vi "Review Results.vi"(0 "Cal Results":string, 5 "Request Message":string, 9 "Request Header":string, 11 "error in (no error)":errorcluster) -> (4 "Response":string, 15 "error out":errorcluster)   [LabVIEW 2023, in "RFCalAndFixtureCharact.Common.lvlib"]
uses:
  RFCalAndFixtureCharact.Common.lvlib
  C:/srd-semi-rfcal-software/AuxTools/STSRFFixtureCharactUtility/Source/Code Modules/Dependencies/NationalInstruments.RFCalibration.ExecutionEngine.dll
  Dependencies/NationalInstruments.RFCalibration.ExecutionEngine.dll
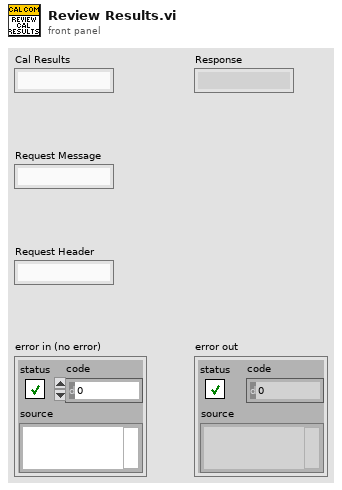
[diagram p1: front panel]
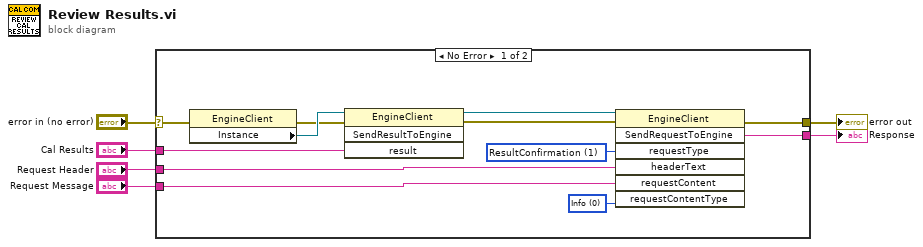
[diagram p0: block diagram]
diagram:
  n1 = case shown="No Error" "error in (no error)" {
    selector: "error in (no error)" -> [w16 w19]
    tunnel: [w18 w19] -> w6
    tunnel: [w17 _] -> w5
    tunnel: "Request Header" -> [w15 _]
    tunnel: "Request Message" -> [w14 _]
    tunnel: "Cal Results" -> [w10 _]
    frame No Error {
      w7 = 0 items=["Info", "Warning", "Error", "Action"] ("requestContentType")
      w8 = 1 items=["Command", "ResultConfirmation", "CheckListenerStatus", "IntermediateResultReview"] ("Request Type")
      n2 = property class="EngineClient"(error in=w16) -> (error out=w9:errorcluster, "Instance"=w13:refnum<k24>)  [unwired: 1 in, 1 out]
      n3 = invoke class="EngineClient" method="SendResultToEngine"(reference=w13, error in=w9, "result"=w10) -> (reference out=w12:refnum<k24>, error out=w11:errorcluster)  [unwired: 1 in, 2 out]
      n4 = invoke class="EngineClient" method="SendRequestToEngine"(reference=w12, error in=w11, "requestType"=w8, "headerText"=w15, "requestContent"=w14, "requestContentType"=w7) -> (error out=w18:errorcluster, "SendRequestToEngine"=w17:string)  [unwired: 1 in, 5 out]
    }
    frame Error {
    }
  }
  "error out" <- w6
  "Response" <- w5
